vi "Drive_Test_PIDs_2.vi"(7 "iterate?":bool) -> (4 "P":dbl=0.0010000000000000002, 15 "goal angle":dbl=190.0)   [LabVIEW 2019]
panel:
  in  "Initial P":dbl=0.0001
  in  "End P":dbl=0.001
  in  "deltaP":dbl=0.0001
  in  "deltaGoal (degrees)":dbl=90.0
  in  "initialAngle (degrees)":dbl
  in  "STOP":bool
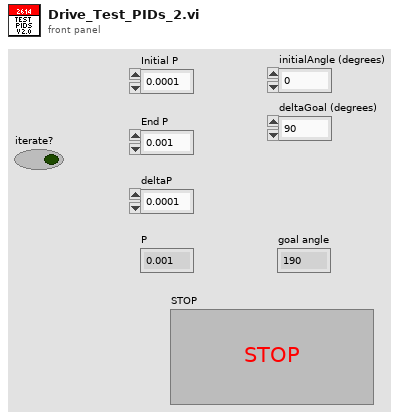
[diagram p1: front panel]
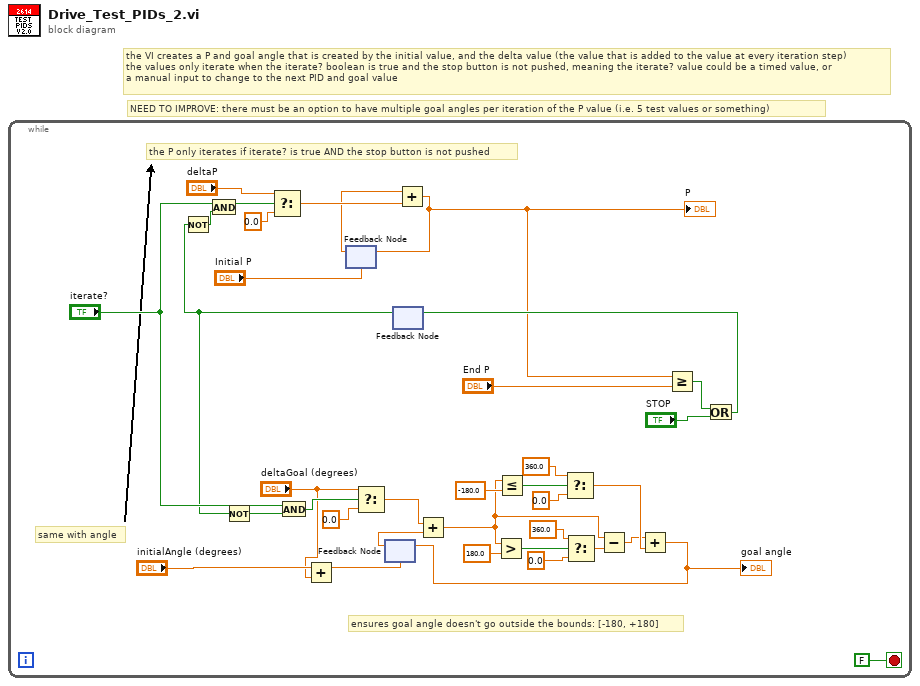
[diagram p0: block diagram]
diagram:
  # "NEED TO IMPROVE: there must be an option to have multiple goal angles per iteration of the P value (i.e. 5 test values or something)"
  # "the VI creates a P and goal angle that is created by the initial value, and the delta value (the value that is added to the value at every iteration step)\nthe values only iterate when the iterate? boolean is true and the stop button is not pushed, meaning the iterate? value could be a timed value, or \na manual input to change to the next PID and goal value"
  n1 = while {
    stop <- FALSE stop-if-true
    # "same with angle"
    # "the P only iterates if iterate? is true AND the stop button is not pushed"
    # "ensures goal angle doesn't go outside the bounds: [-180, +180]"
    n2 = Add(x="initialAngle (degrees)", y="deltaGoal (degrees)") -> (x+y=w2:dbl)
    n3 = feedback #1("Initial P") -> (w20:dbl)
    n4 = feedback #2(w2) -> (w29:dbl)
    n5 = feedback #3() -> (w30:bool)  [unwired: 1 in]
    n6 = Not(x=w30) -> (.not. x?=w27:bool)
    n7 = And(x="iterate?", y=w27) -> (x .and. y?=w25:bool)
    n8 = Not(x=w30) -> (.not. x?=w31:bool)
    n9 = Select(t="deltaP", s=w25, f=0.0) -> (s? t:f=w23:dbl)
    n10 = And(x="iterate?", y=w31) -> (x .and. y?=w33:bool)
    n11 = Select(t="deltaGoal (degrees)", s=w33, f=0.0) -> (s? t:f=w35:dbl)
    n12 = Add(x=w20, y=w23) -> (x+y=w24:dbl)
    "P" <- w24
    n13 = feedback-in #1(w24) -> ()
    n14 = Add(x=w35, y=w29) -> (x+y=w11:dbl)
    n15 = Greater?(x=w11, y=180.0) -> (0:w8:bool)
    n16 = Less Or Equal?(x=w11, y=-180.0) -> (x <= y?=w14:bool)
    n17 = Select(t=360.0, s=w14, f=0.0) -> (s? t:f=w18:dbl)
    n18 = Select(t=360.0, s=w8, f=0.0) -> (s? t:f=w10:dbl)
    n19 = Subtract(x=w11, y=w10) -> (x-y=w17:dbl)
    n20 = Add(x=w17, y=w18) -> (x+y=w36:dbl)
    "goal angle" <- w36
    n21 = feedback-in #2(w36) -> ()
    n22 = Greater Or Equal?(x=w24, y="End P") -> (x >= y?=w6:bool)
    n23 = Or(x=w6, y="STOP") -> (x .or. y?=w26:bool)
    n24 = feedback-in #3(w26) -> ()
  }
